vi "UMB_scaleGoodness.vi"(1 "goodness":dbl[](array[numeric])) -> (0 "scaled goodness":dbl[](array[numeric]))   [LabVIEW 2012]
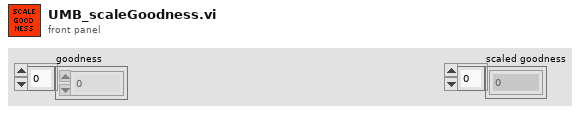
[diagram p1: front panel]
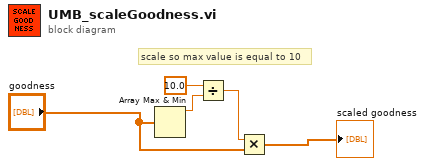
[diagram p0: block diagram]
diagram:
  # "scale so max value is equal to 10"
  n1 = Array Max & Min(array="goodness") -> (max value=w4:dbl)  [unwired: 3 out]
  n2 = Divide(x=10.0, y=w4) -> (x/y=w3:dbl)
  n3 = Multiply(x=w3, y="goodness") -> (x*y=→"scaled goodness":dbl[])
